vi "Get sensor polarity (SubVI).vi"(11 "R вх":dbl) -> (4 "R по модулю":dbl format="%#.1g", 10 "Цвет полярности вкл. R":u32)   [LabVIEW 2015]
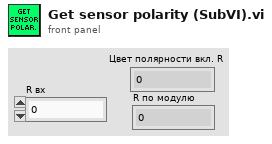
[diagram p1: front panel]
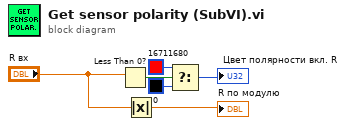
[diagram p0: block diagram]
diagram:
  n1 = Less Than 0?(x="R вх") -> (x < 0?=w5:bool)
  n2 = Absolute Value(x="R вх") -> (abs(x)=→"R по модулю":dbl)
  n3 = Select(t=u32 16711680, s=w5, f=u32 0) -> (s? t:f=→"Цвет полярности вкл. R":u32)
